vi "Analyze Filter Banks.vi"() -> ()   [LabVIEW 2023]
doc: "This example demonstrates how to use the <b>DFD Plot Filter Bank Frequency Response</b> VI and the <b>DFD Analyze Filter Bank Distortion</b> VI to analyze a filter bank.\n\nComplete the following steps to use this VI:\n1) Run this VI.\n2) On the <b>Frequency Responses</b> tab, observe the magnitude and phase responses of the filter bank.\n3) On the <b>Distortions</b> tab, observe the aliasing, magnitude distortion, and phase distortion in the filter bank.\n4) Change the filter bank specifications and observe the characteristics of the new filter bank. If <b>PR?</b> is TRUE, the aliasing is negligible, the magnitude distortion is small, and the phase is linear."
uses:
  <vilib>/addons/Digital Filter Design/_Objects.llb/DFD Phase Setting.ctl
  <vilib>/addons/Digital Filter Design/NI_DigFilter_FilterBank.lvlib
  <vilib>/addons/Digital Filter Design/NI_DigFilterLicensed.lvlib
panel:
  out "Error Message":string
  in  "PR?":bool
  in  "Tab Control":enum32{"Frequency Responses", "Distortions"}(tab)
  out "Magnitude Responses":cluster{"Y":dbl[], "Y":dbl[]}[](graph)
  out "Phase Responses":cluster{"Y":dbl[], "Y":dbl[]}[](graph)
  out "Aliasing":cluster{dbl[], "values":dbl[]}(graph)
  out "Magnitude Distortion":cluster{dbl[], "values":dbl[]}(graph)
  out "Phase Distortion":cluster{dbl[], "values":dbl[]}(graph)
  in  "#Bands":i32=4
  in  "Order":i32=39
  in  "Roll Off":dbl=0.2 min=0.0001 max=0.9999
  in  "Weight":dbl=0.5 min=0.0 max=1.0
  in  "dB on?":bool=TRUE
  in  "Phase View":T1={"unwrap? (F)"=TRUE, "degree? (F)"=FALSE}
  in  "stop 2":bool
  # "Select Help>>Show Context Help and move the cursor over the VI icon for more information."
  # "Specifications"
  # "Display Settings"
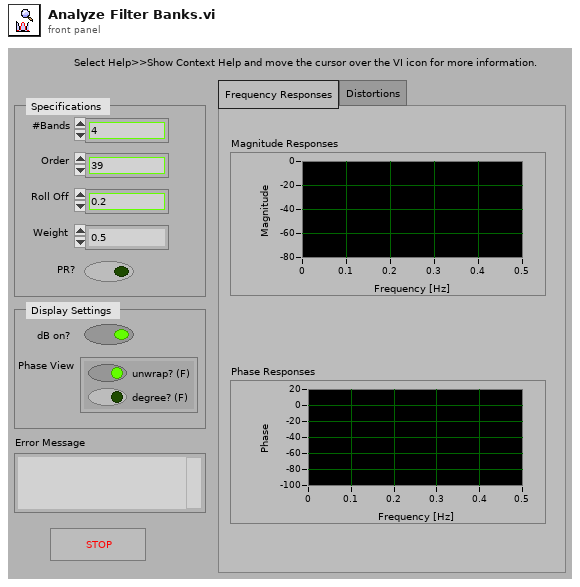
[diagram p1: front panel]
types:
  T1 = typedef "NI_DigFilterLicensed.lvlib/DFD Phase Setting.ctl" = cluster{"unwrap? (F)":bool, "degree? (F)":bool}
  T2 = typedef "NI_DigFilter_FilterBank.lvlib/DFD Filter Bank Obj.ctl" = cluster{"mFBank_AnalysisFilters":T3[], "mFBank_SynthesisFilters":T3[], "mFBank_#Bands":i32, "mFBank_ProcMethod":T8, "mFBank_Coeffs":dbl[], "mFBank_Gain":dbl, "mFBank_Delay":i32, "mFBank_Type":T9}
  T3 = typedef "NI_DigFilterLicensed.lvlib/DFD Multirate Filter Obj.ctl" = cluster{"mMRate_Structure":enum16{"CIC", "FIR", "IIR", "Lattice"}, "mMRate_Mode":T4, "mMRate_Factor":i32, "mMRate_FIRParams":cluster{"mMRate_FIR_H":dbl[], "mMRate_FIR_IsNyquist?":bool, "mMRate_FIR_IsSymmetric?":bool}, "mMRate_CICParams":cluster{"mMRate_CIC_#Stage":i32, "mMRate_CIC_Lag":i32, "mMRate_CIC_Type":enum16{"Lowpass", "Highpass"}}, "mMRate_Order":i32, "mMRate_Version":string, "mMRate_Comments":string, "mMRate_RationalFactor":cluster{"mMRate_L":i32, "mMRate_M":i32}, "mMRate_Fs":dbl, "mMRate_Quantized?":bool, "mMRate_QFilterGain":dbl, "mMRate_CoefWl":i16, "mMRate_Scaling":cluster{"mMRate_ScaleByPowerOf2?":bool, "mMRate_ScaleType":T5}, "mMRate_InputWl":i16, "mMRate_OutputWl":i16, "mMRate_OutputMode":T6, "mMRate_MultMode":T7, "mMRate_BitPruning":bool, "mMRate_GainWl":i16, "mMRate_OutputFwl":i16, "mMRate_SumIwl":i16, "mMRate_InputIwl ":i16, "mMRate_SumWl":i16, "mMRate_CoefIwl":i16}
  T4 = typedef "NI_DigFilterLicensed.lvlib/DFD Multirate Mode.ctl" = i16
  T5 = typedef "NI_DigFilterLicensed.lvlib/DFD Coef Norm Type.ctl" = enum16{"No Norm", "Time Domain 1-Norm", "Time Domain 2-Norm", "Time Domain Inf-Norm"}
  T6 = typedef "NI_DigFilterLicensed.lvlib/DFD Round-off Mode.ctl" = enum16{"Nearest", "Truncation"}
  T7 = typedef "NI_DigFilterLicensed.lvlib/DFD FXP MRate Multiply Mode.ctl" = enum16{"Truncated", "Full"}
  T8 = typedef "NI_DigFilter_FilterBank.lvlib/DFD Filter Bank Processing Method.ctl" = enum16{"General", "2-Band QMF Lattice", "Cosine-Modulated"}
  T9 = typedef "NI_DigFilter_FilterBank.lvlib/DFD Filter Bank Type.ctl" = u16
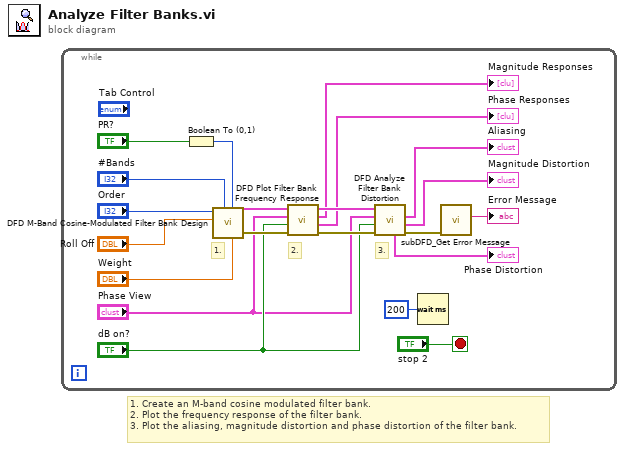
[diagram p0: block diagram]
diagram:
  # "1. Create an M-band cosine modulated filter bank.\n2. Plot the frequency response of the filter bank.\n3. Plot the aliasing, magnitude distortion and phase distortion of the filter bank."
  n1 = while {
    stop <- "stop 2" stop-if-true
    # "3."
    # "2."
    # "1."
    n2 = Boolean To (0,1)(Boolean="PR?") -> (0, 1=w8:i16)
    n3 = call <vilib>:"DFD M-Band Cosine-Modulated Filter Bank Design.vi"("weight"="Weight", "signal reconstruction"=w8, "band counts"="#Bands", "roll off"="Roll Off", "order"="Order") -> ("error out"=w18:errorcluster, "filter bank out"=w19:T2)  [unwired: 5 in]
    n4 = call <vilib>:"DFD Plot Filter Bank Frequency Response.vi"("error in (no error)"=w18, "dB on? (T)"="dB on?", "phase view"="Phase View", "filter bank in"=w19) -> ("error out"=w20:errorcluster, "phase responses"=→"Phase Responses":cluster{"Y":dbl[], "Y":dbl[]}[], "magnitude responses"=→"Magnitude Responses":cluster{"Y":dbl[], "Y":dbl[]}[], "filter bank out"=w12:T2)  [unwired: 4 in]
    n5 = call <vilib>:"DFD Analyze Filter Bank Distortion.vi"("error in (no error)"=w20, "dB on? (T)"="dB on?", "phase view"="Phase View", "filter bank in"=w12) -> ("error out"=w7:errorcluster, "magnitude distortion"=→"Magnitude Distortion":cluster{dbl[], "values":dbl[]}, "aliasing"=→"Aliasing":cluster{dbl[], "values":dbl[]}, "phase distortion"=→"Phase Distortion":cluster{dbl[], "values":dbl[]})  [unwired: 3 in, 1 out]
    n6 = Wait (ms)(milliseconds to wait=u32 200) -> ()  [unwired: 1 out]
    n7 = call <vilib>:"subDFD_Get Error Message.vi"("error in (no error)"=w7) -> ("Error Message"=→"Error Message":string)  [unwired: 10 in]
  }
